vi "AlphaBetaToABC_PowInv.vi"(0 "alpha":sgl format="%#_32g", 5 "beta":sgl format="%#_32g", 12 "Resources":T1) -> (4 "A":sgl format="%#_32g", 6 "B":sgl, 8 "C":sgl)   [LabVIEW 2017]
uses:
  Multiplier/Multiplier.lvclass
  Adder/Adder.lvclass
  Subtractor/Subtractor.lvclass
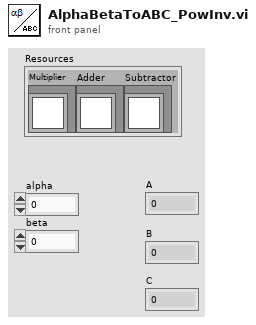
[diagram p1: front panel]
types:
  T1 = cluster{"Multiplier":refnum<class "Multiplier.lvclass">, "Adder":refnum<class "Adder.lvclass">, "Subtractor":refnum<class "Subtractor.lvclass">}
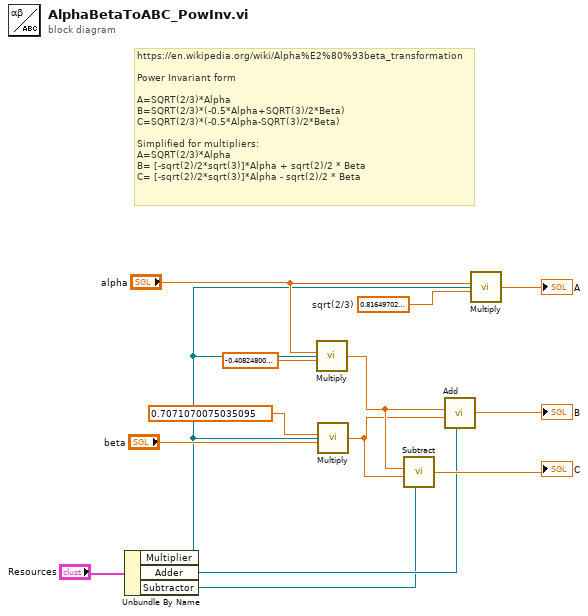
[diagram p0: block diagram]
diagram:
  w10 = sgl 0.816497  # sqrt(2/3)
  # "https://en.wikipedia.org/wiki/Alpha%E2%80%93beta_transformation\n\nPower Invariant form\n\nA=SQRT(2/3)*Alpha\nB=SQRT(2/3)*(-0.5*Alpha+SQRT(3)/2*Beta)\nC=SQRT(2/3)*(-0.5*Alpha-SQRT(3)/2*Beta)\n\nSimplified for multipliers:\nA=SQRT(2/3)*Alpha\nB= [-sqrt(2)/2*sqrt(3)]*Alpha + sqrt(2)/2 * Beta\nC= [-sqrt(2)/2*sqrt(3)]*Alpha - sqrt(2)/2 * Beta"
  n1 = Unbundle By Name("Resources") -> ("Multiplier"=w3:refnum<class "Multiplier.lvclass">, "Adder"=w2:refnum<class "Adder.lvclass">, "Subtractor"=w1:refnum<class "Subtractor.lvclass">)
  n2 = call-dynamic "Multiply.vi"("x"="alpha", "y"=sgl -0.408248, "Multiplier"=w3) -> ("x*y"=w7:sgl)  [unwired: 4 in]
  n3 = call-dynamic "Multiply.vi"("x"=sgl 0.707107 ("beta"), "y"="beta", "Multiplier"=w3) -> ("x*y"=w6:sgl)  [unwired: 4 in]
  n4 = call-dynamic "Subtract.vi"("x"=w7, "y"=w6, "Subtractor"=w1) -> ("x-y"=→"C":sgl)  [unwired: 4 in]
  n5 = call-dynamic "Add.vi"("x"=w7, "y"=w6, "Adder"=w2) -> ("x+y"=→"B":sgl)  [unwired: 4 in]
  n6 = call-dynamic "Multiply.vi"("x"="alpha", "y"=w10, "Multiplier"=w3) -> ("x*y"=→"A":sgl)  [unwired: 4 in]
